vi "RT Get Bare Timestamp.vi"() -> (2 "Timestamp":u64)   [LabVIEW 2013]
doc: "Inserts a 64-bit timestamp value from a high-precision timing source into a preallocated array at an index value specified by <B>iteration</B>. The timestamp value indicates the time when the RT Get Timestamp VI executes on the RT target."
uses:
  <vilib>/ni_emb.dll
panel:
  # "Just get timestamp as U64 w/o storing anywhere."
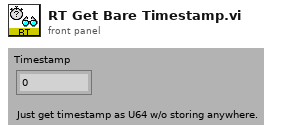
[diagram p1: front panel]
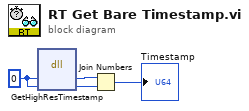
[diagram p0: block diagram]
diagram:
  w3 = u32 0 ("InH")
  n1 = dll-call lib="C:/Program Files (x86)/National Instruments/LabVIEW 2013/Targets/NI/RT/vi.lib/ni_emb.*" fn="GetHighResTimestamp"("tsH"=w3, "tsL"=w3) -> ("tsH"=w2:u32, "tsL"=w1:u32)  [unwired: 3 in, 3 out]
  n2 = Join Numbers(hi=w2, lo=w1) -> ((hi.lo)=→"Timestamp":u64)
